vi "SAC-Enum Data Files.vi"(0 "State":T1, 7 "Azimuths":dbl[](array[numeric]), 11 "ASTFs":bool) -> (4 "filestems":string[](array[string]), 8 "file status":bool[](array[boolean]))   [LabVIEW 2020]
uses:
  Typedefs/SAC-State.ctl
  <vilib>/regexp/Match Regular Expression.xnode
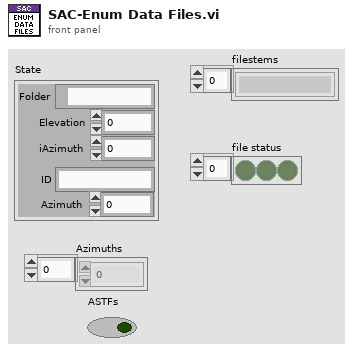
[diagram p1: front panel]
types:
  T1 = typedef "SAC-State.ctl" = cluster{"Folder":path, "Elevation":dbl, "iAzimuth":i32, "ID":string, "Azimuth":dbl}
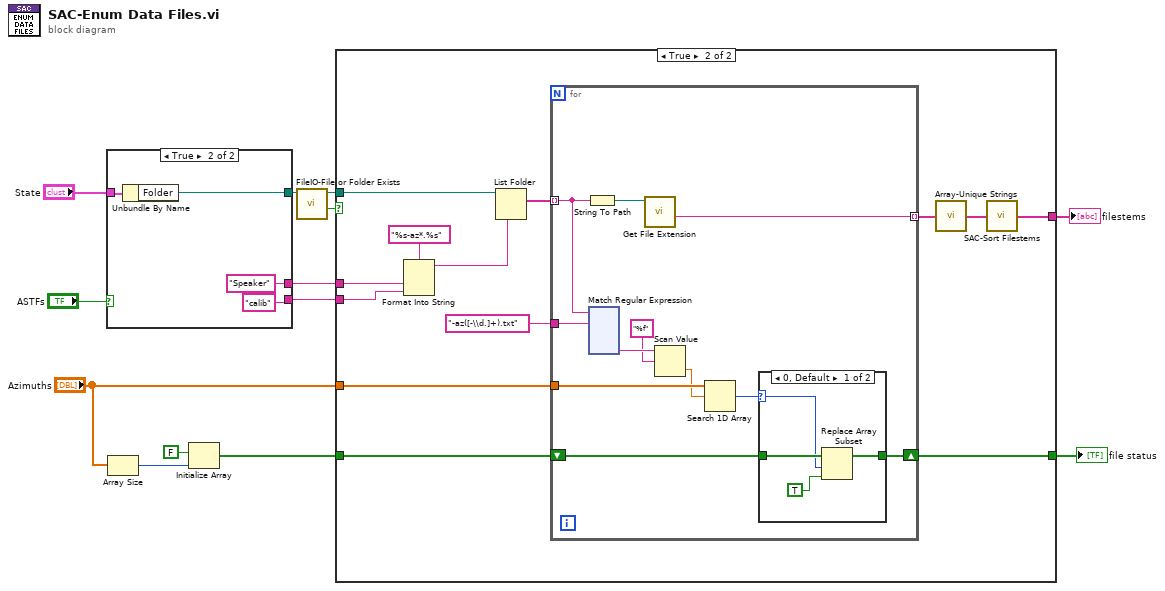
[diagram p0: block diagram]
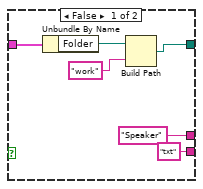
[diagram p2: hidden frame]
diagram:
  n1 = case shown="True" "ASTFs" {
    tunnel: ["Speaker" "Speaker"] -> w13
    tunnel: ["txt" "calib"] -> w4
    tunnel: "State" -> [w18 w21]
    tunnel: [w16 w20] -> w1
    frame False {
      n2 = Unbundle By Name(w18) -> ("Folder"=w17:path)
      n3 = Build Path(base path=w17, name or relative path="work") -> (appended path=w16:path)
    }
    frame True {
      n4 = Unbundle By Name(w21) -> ("Folder"=w20:path)
    }
  }
  n5 = Array Size(array="Azimuths") -> (size(s)=w5:i32)
  n6 = Initialize Array(FALSE, w5) -> (w11:bool[])
  n7 = call "FileIO-File or Folder Exists.vi"("path"=w1) -> ("Exists?"=w6:bool, "dup path"=w7:path)  [unwired: 7 in, 2 out]
  n8 = case shown="True" w6 {
    tunnel: w13 -> [_ w36]
    tunnel: w7 -> [_ w35]
    tunnel: w11 -> [w24 w32]
    tunnel: "Azimuths" -> [_ w31]
    tunnel: [w24 w29] -> w9
    tunnel: [_ w25] -> w8
    tunnel: w4 -> [_ w27]
    frame False {
    }
    frame True {
      n9 = Format Into String(format string="%s-az*.%s", w36, w27) -> (resulting string=w34:string)  [unwired: 2 in, 1 out]
      n10 = List Folder(path=w35, pattern=w34) -> (filenames=w33:string[])  [unwired: 2 in, 3 out]
      n11 = for {
        tunnel: w33 -> [w40] mode=indexing
        shift-right: [w44] -> w29
        shift-left: w32 -> [w45]
        tunnel: w31 -> [w47]
        tunnel: "-az([-\\d.]+).txt" ("regular expression") -> [w48]
        tunnel: [w38] -> w28 mode=indexing
        n12 = String To Path(string=w40) -> (path=w39:path)
        n13 = xnode "Match Regular Expression"("input string"=w40, "regular expression"=w48) -> ("submatch 1"=w42:string)  [unwired: 4 in, 5 out]
        n14 = call <vilib>:"Get File Extension.vi"("file"=w39) -> ("filename without extension"=w38:string)  [unwired: 6 in, 4 out]
        n15 = Scan Value(string=w42, format string="%f") -> (value=w46:dbl)  [unwired: 1 in, 1 out]
        n16 = Search 1D Array(1D array=w47, element=w46) -> (index of element=w43:i32)  [unwired: 1 in]
        n17 = case shown="0, Default" w43 {
          selector: w43 -> [w49 _]
          tunnel: w45 -> [w52 w53]
          tunnel: [w51 w53] -> w44
          frame 0, Default {
            n18 = Replace Array Subset(array=w52, new element=TRUE ("new element/subarray"), index=w49) -> (w51:bool[])
          }
          frame -1 {
          }
        }
      }
      n19 = call "Array-Unique Strings.vi"("Strings"=w28) -> ("Unique strings"=w26:string[])  [unwired: 4 in]
      n20 = call "SAC-Sort Filestems.vi"("Filestems"=w26) -> ("Sorted filestems"=w25:string[])  [unwired: 14 in]
    }
  }
  "file status" <- w9
  "filestems" <- w8
